vi "Autonomous Independent.vi"() -> ()   [LabVIEW 2016]
doc: "This VI is called when autonomous begins, and will automatically be terminated when autonomous ends. You can carry out timed or sensor driven robot movement independently without needing to return to the caller."
uses:
  <vilib>/Rock Robotics/WPI/Solenoid/WPI_SolenoidValue.ctl
  <vilib>/Rock Robotics/Network Tables/NT Read String.vi
  Robot Global Data.vi
  <vilib>/Rock Robotics/WPI/Solenoid/WPI_SolenoidSetEnum.vi
  <vilib>/Rock Robotics/WPI/Utilities/WPI_GetSetVariantRefNum.vi
  <vilib>/addons/control/pid/pid.llb/PID (DBL).vi
  <vilib>/addons/control/pid/NI_PID_pid.lvlib
panel:
  in  "Center":dbl=180.0 format="%#_13g"
  in  "MOE":dbl=25.0 format="%#_13g"
  in  "Speed 2":dbl=0.45 format="%#_13g"
  in  "PID gains L":T1={"proportional gain (Kc)"=1.5e-05, "integral time (Ti, min)"=1e-07, "derivative time (Td, min)"=0.0} {"derivative time (Td, min)" format="%.3f"; "integral time (Ti, min)" format="%.6f"; "proportional gain (Kc)" format="%.6f"}
  in  "PID gains R":T1={"proportional gain (Kc)"=1.5e-05, "integral time (Ti, min)"=1e-07, "derivative time (Td, min)"=0.0} {"derivative time (Td, min)" format="%.3f"; "integral time (Ti, min)" format="%.6f"; "proportional gain (Kc)" format="%.6f"}
  in  "Range":cluster{"output high":dbl, "output low":dbl}={"output high"=1.0, "output low"=-1.0} {"output low" format="%.2f"; "output high" format="%.2f"}
  out "Right V":cluster{"output":dbl, dbl, "Numeric":dbl}(graph)
  out "Left V":cluster{"output":dbl, dbl, "Numeric":dbl}(graph)
  in  "Speed":dbl=1.0 format="%#_13g"
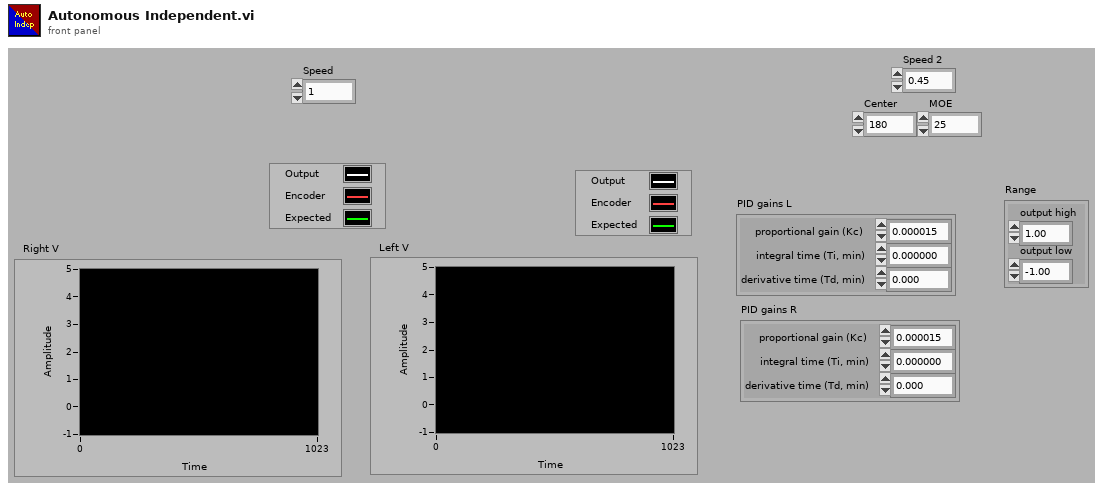
[diagram p1: front panel]
types:
  T1 = cluster{"proportional gain (Kc)":dbl, "integral time (Ti, min)":dbl, "derivative time (Td, min)":dbl}
  T2 = typedef "WPI_SolenoidValue.ctl" = enum16{"Off", "On", "Forward", "Reverse"}
  T3 = typedef "WPI_SolenoidDevRef.ctl" = cluster{"DevStatus":errorcluster, "Pneumatics Control Module":u8, "Forward Solenoid Channel":T4, "Reverse Solenoid Channel":T4}
  T4 = typedef "WPI_SolenoidChannel.ctl" = enum8{"Solenoid 0", "Solenoid 1", "Solenoid 2", "Solenoid 3", "Solenoid 4", "Solenoid 5", "Solenoid 6", "Solenoid 7", "Invalid"}
  T5 = typedef "WPI_RobotDriveDevRef.ctl" = cluster{"DevStatus":errorcluster, "Motors[]":T6[], "Square Inputs":bool, "Max Output":dbl}
  T6 = typedef "WPI_MotorControlDeviceRef.ctl" = cluster{"DeviceStatus":errorcluster, "Type":T7, "PWM":cluster{"PWM Channel":T8, "DeadBand":T9}, "CAN":cluster{"Device Number":u8, "SetOutput VI Ref":variant, "GetOutput VI Ref":variant, "Enable VI Ref":variant, "Disable VI Ref":variant, "Data":variant}, "Invert":bool}
  T7 = typedef "WPI_MotorControlType.ctl" = enum16{"PWM", "CAN"}
  T8 = typedef "FPGA_DIOPWMChannel.ctl" = enum8{"PWM 0", "PWM 1", "PWM 2", "PWM 3", "PWM 4", "PWM 5", "PWM 6", "PWM 7", "PWM 8", "PWM 9", "PWM MXP 0", "PWM MXP 1", "PWM MXP 2", "PWM MXP 3", "PWM MXP 4", "PWM MXP 5", "PWM MXP 6", "PWM MXP 7", "PWM MXP 8", "PWM MXP 9", "Invalid"}
  T9 = typedef "WPI_PWMDeadband.ctl" = cluster{"Name":string, "maxPositivePwm":i32, "minPositivePwm":i32, "centerPwm":i32, "maxNegativePwm":i32, "minNegativePwm":i32, "angularRange":u16}
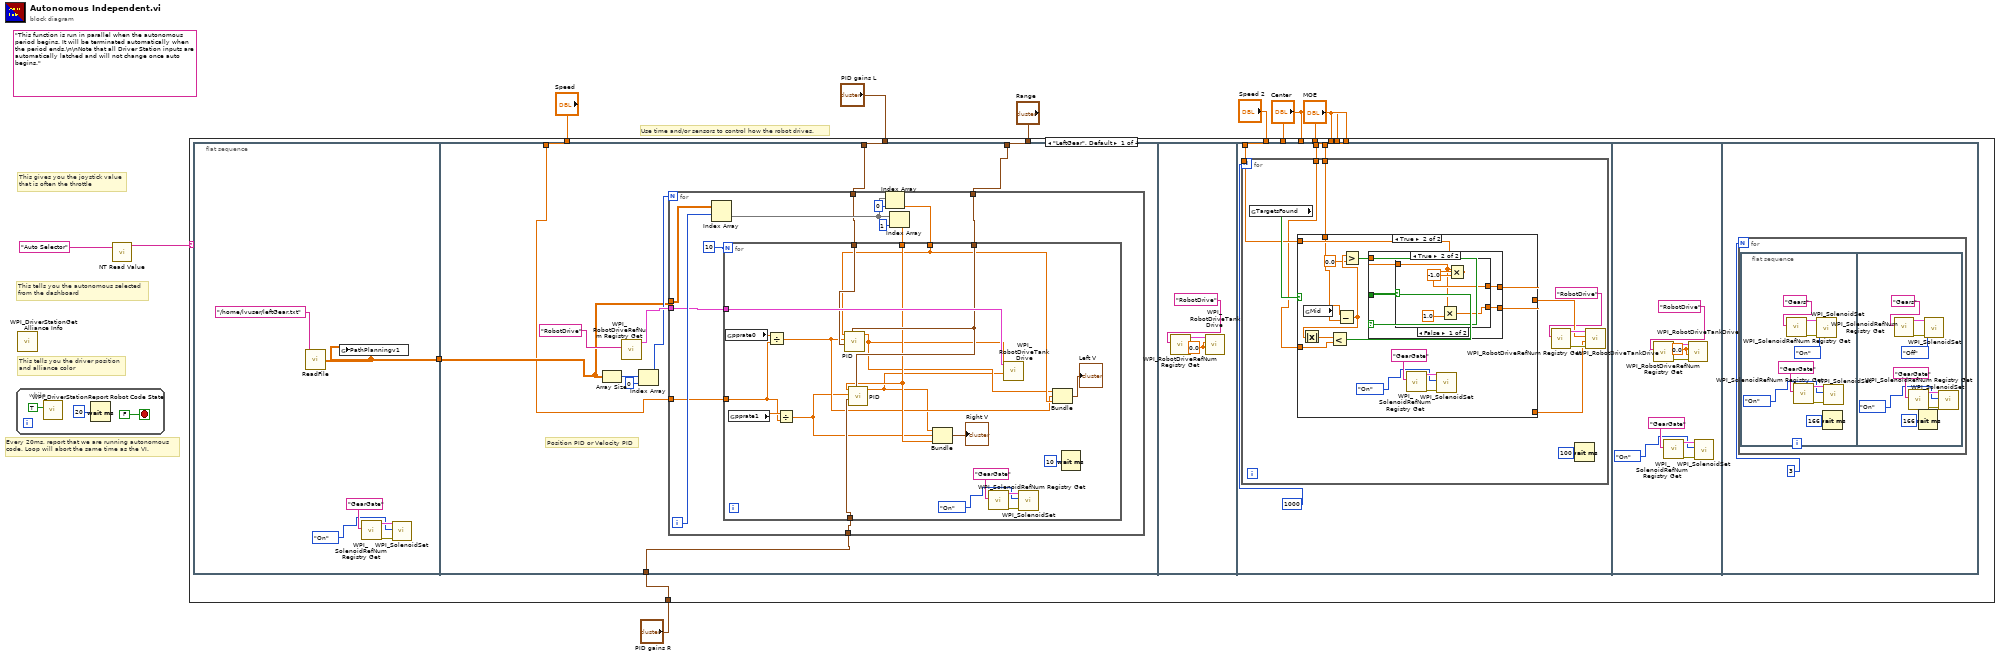
[diagram p0: block diagram]
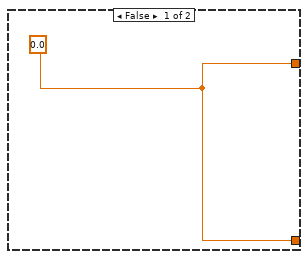
[diagram p2: hidden frame]
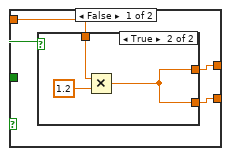
[diagram p3: hidden frame]
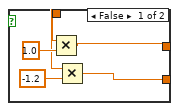
[diagram p4: hidden frame]
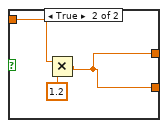
[diagram p5: hidden frame]
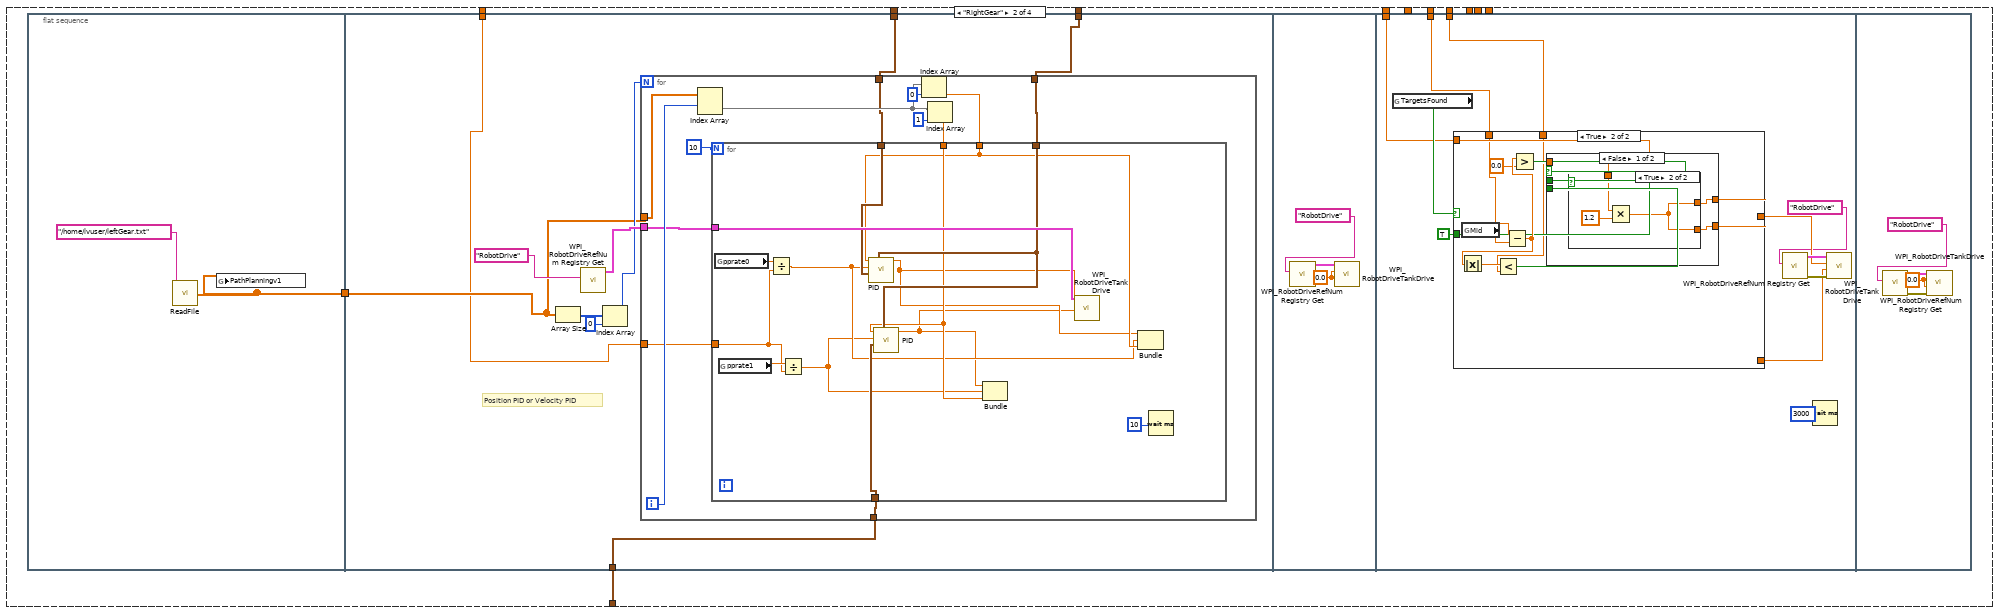
[diagram p6: hidden frame]
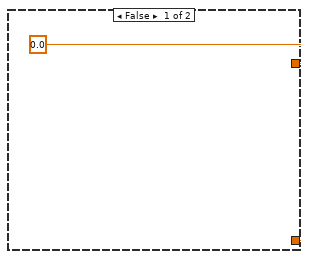
[diagram p7: hidden frame]
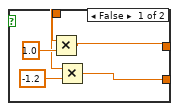
[diagram p8: hidden frame]
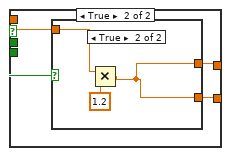
[diagram p9: hidden frame]
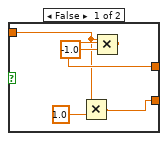
[diagram p10: hidden frame]
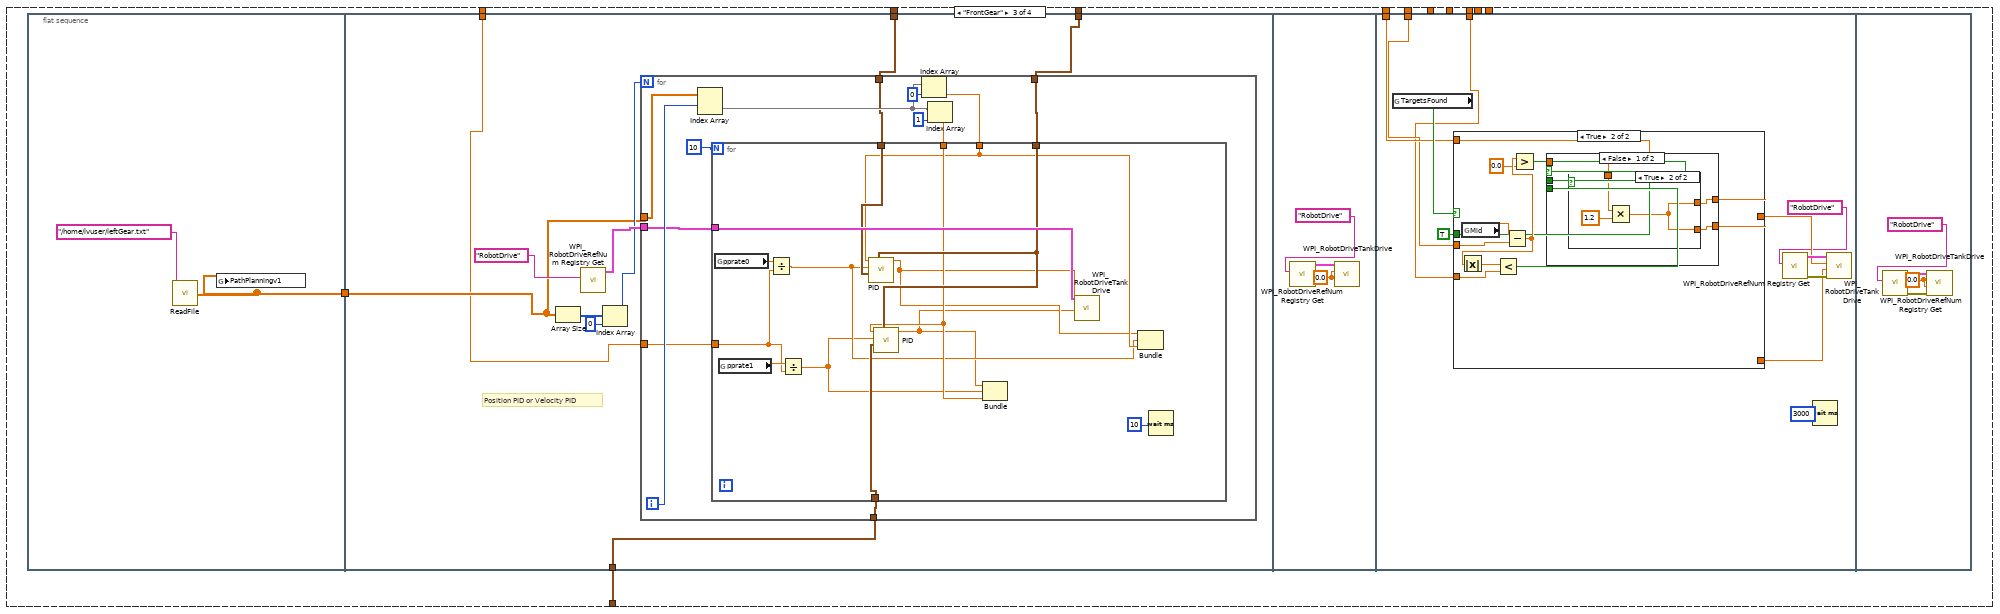
[diagram p11: hidden frame]
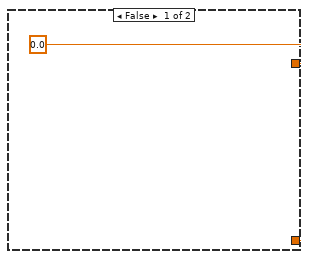
[diagram p12: hidden frame]
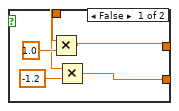
[diagram p13: hidden frame]
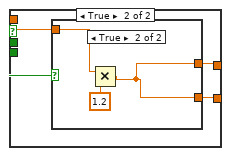
[diagram p14: hidden frame]
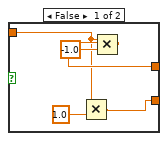
[diagram p15: hidden frame]
diagram:
  (unwired) "This function is run in parallel when the autonomous period begins. It will be terminated automatically when the period ends.\n\nNote that all Driver Station inputs are automatically latched and will not change once auto begins."
  # "This tells you the autonomous selected\nfrom the dashboard"
  # "Every 20ms, report that we are running autonomous\ncode. Loop will abort the same time as the VI."
  # "This gives you the joystick value\nthat is often the throttle"
  # "Use time and/or sensors to control how the robot drives."
  # "This tells you the driver position\nand alliance color"
  n1 = while {
    stop <- FALSE stop-if-true
    n2 = call <vilib>:"WPI_DriverStationReport Robot Code State.vi"("Autonomous"=TRUE) -> ()  [unwired: 10 in, 1 out]
    n3 = Wait (ms)(milliseconds to wait=u32 20) -> ()  [unwired: 1 out]
  }
  n4 = call <vilib>:"WPI_DriverStationGet Alliance Info.vi"() -> ()  [unwired: 12 out]
  n5 = call-poly <vilib>:"NT Read Value.vi"("Name"="Auto Selector") -> ("String"=w8:string)  [unwired: 9 in, 1 out]
  n6 = case shown="\"LeftGear\", Default" w8 {
    tunnel: "Range" -> [w19 w160 w262 _]
    tunnel: "PID gains L" -> [w18 w159 w261 _]
    tunnel: "Speed 2" -> [w17 w157 w260 _]
    tunnel: "Center" -> [w16 _ _ _]
    tunnel: "MOE" -> [w15 _ _ _]
    tunnel: "Speed" -> [w14 w158 w257 _]
    tunnel: "Center" -> [_ w156 _ _]
    tunnel: "MOE" -> [_ w155 _ _]
    tunnel: "Center" -> [_ _ w259 _]
    tunnel: "MOE" -> [_ _ w258 _]
    tunnel: "PID gains R" -> [w13 w154 w256 _]
    frame "LeftGear", Default {
      n7 = flat-sequence {
        tunnel: [w25] -> w20
        tunnel: w20 -> [w31]
        tunnel: w19 -> [w30]
        tunnel: w18 -> [w29]
        tunnel: w14 -> [w28]
        tunnel: w13 -> [w27]
        tunnel: w17 -> [w76]
        tunnel: w16 -> [w75]
        tunnel: w15 -> [w74]
        frame #0 {
          n8 = call "ReadFile.vi"("Name"="/home/lvuser/leftGear.txt") -> ("Array - Numeric"=w25:dbl[][])
          n9 = global write "Robot Global Data.vi" "PathPlanningv1"(w25) -> ()
          n10 = call <vilib>:"WPI_SolenoidRefNum Registry Get.vi"("refnum name"="GearGate") -> ("error out"=w24:errorcluster, "SolenoidDevRef"=w23:T3)  [unwired: 9 in]
          n11 = call-poly <vilib>:"WPI_SolenoidSet.vi"("error in (no error)"=w24, "Value"=WPI_SolenoidValue."On", "SolenoidDevRef"=w23) -> ()  [unwired: 7 in, 2 out]
        }
        frame #1 {
          # "Position PID or Velocity PID"
          n12 = Array Size(array=w31) -> (size(s)=w36:i32[])
          n13 = call <vilib>:"WPI_RobotDriveRefNum Registry Get.vi"("refnum name"="RobotDrive") -> ("RobotDriveDevRef"=w33:T5)  [unwired: 9 in, 1 out]
          n14 = Index Array(array=w36, index=0) -> (element=w32:i32)
          n15 = for {
            N: w32 -> [_]
            tunnel: w31 -> [w46]
            tunnel: w27 -> [w41]
            tunnel: w29 -> [w40]
            tunnel: w30 -> [w39]
            tunnel: w33 -> [w38]
            tunnel: w28 -> [w37]
            i -> [w43]
            n16 = Index Array(array=w46, index (row)=w43) -> (element=w49:dbl[])  [unwired: 1 in]
            n17 = Index Array(array=w49, index=0) -> (element=w45:dbl)
            n18 = Index Array(array=w49, index=1) -> (element=w44:dbl)
            n19 = for {
              N: 10 -> [_]
              tunnel: w45 -> [w63]
              tunnel: w44 -> [w64]
              tunnel: w41 -> [w67]
              tunnel: w40 -> [w66]
              tunnel: w39 -> [w65]
              tunnel: w38 -> [w68]
              tunnel: w37 -> [w56]
              n20 = global read "Robot Global Data.vi" "pprate0"() -> (w60:dbl)
              n21 = global read "Robot Global Data.vi" "pprate1"() -> (w57:dbl)
              n22 = Divide(x=w60, y=w56) -> (x/y=w59:dbl)
              n23 = Divide(x=w57, y=w56) -> (x/y=w58:dbl)
              n24 = call-poly <vilib>:"PID.vi"("output range"=w65, "PID gains"=w66, "process variable"=w59, "setpoint"=w63) -> ("output"=w55:dbl)  [unwired: 6 in, 1 out]
              n25 = call-poly <vilib>:"PID.vi"("output range"=w65, "PID gains"=w67, "process variable"=w58, "setpoint"=w64) -> ("output"=w54:dbl)  [unwired: 6 in, 1 out]
              n26 = Bundle("output"=w54, w58, "Numeric"=w64) -> (→"Right V":cluster{"output":dbl, dbl, "Numeric":dbl})  [unwired: 1 in]
              n27 = call <vilib>:"WPI_SolenoidRefNum Registry Get.vi"("refnum name"="GearGate") -> ("error out"=w53:errorcluster, "SolenoidDevRef"=w52:T3)  [unwired: 9 in]
              n28 = call <vilib>:"WPI_RobotDriveTankDrive.vi"("Right axis value"=w54, "Left axis value"=w55, "RobotDriveDevRef"=w68) -> ()  [unwired: 6 in, 3 out]
              n29 = call-poly <vilib>:"WPI_SolenoidSet.vi"("error in (no error)"=w53, "Value"=WPI_SolenoidValue."On", "SolenoidDevRef"=w52) -> ()  [unwired: 7 in, 2 out]
              n30 = Bundle("output"=w55, w59, "Numeric"=w63) -> (→"Left V":cluster{"output":dbl, dbl, "Numeric":dbl})  [unwired: 1 in]
              n31 = Wait (ms)(milliseconds to wait=10) -> ()  [unwired: 1 out]
            }
          }
        }
        frame #2 {
          w71 = 0.0 ("Right axis value")
          n32 = call <vilib>:"WPI_RobotDriveRefNum Registry Get.vi"("refnum name"="RobotDrive") -> ("RobotDriveDevRef"=w72:T5)  [unwired: 9 in, 1 out]
          n33 = call <vilib>:"WPI_RobotDriveTankDrive.vi"("Right axis value"=w71, "Left axis value"=w71, "RobotDriveDevRef"=w72) -> ()  [unwired: 6 in, 3 out]
        }
        frame #3 {
          n34 = for {
            N: 1000 -> [_]
            tunnel: w76 -> [w79]
            tunnel: w75 -> [w78]
            tunnel: w74 -> [w77]
            n35 = global read "Robot Global Data.vi" "TargetsFound"() -> (w80:bool)
            n36 = case shown="True" w80 {
              tunnel: [w87 w99] -> w83
              tunnel: [w87 w98] -> w84
              tunnel: w79 -> [_ w94]
              tunnel: w78 -> [_ w93]
              tunnel: w77 -> [_ w92]
              frame False {
                w87 = 0.0
              }
              frame True {
                n37 = global read "Robot Global Data.vi" "Mid"() -> (w102:dbl)
                n38 = Subtract(x=w102, y=w93) -> (x-y=w96:dbl)
                n39 = Absolute Value(x=w96) -> (abs(x)=w101:dbl)
                n40 = Less?(x=w101, y=w92) -> (x < y?=w100:bool)
                n41 = Greater?(x=w96, y=0.0) -> (0:w97:bool)
                n42 = case shown="True" w97 {
                  tunnel: w100 -> [w103 w118]
                  tunnel: [w104 w116] -> w99
                  tunnel: [w105 w117] -> w98
                  tunnel: w94 -> [w106 w115]
                  frame False {
                    n43 = case shown="True" w103 {
                      tunnel: [w111 w114] -> w105
                      tunnel: [w109 w114] -> w104
                      tunnel: w106 -> [w107 w112]
                      frame False {
                        n44 = Multiply(x=w107, y=1.0) -> (x*y=w111:dbl)
                        n45 = Multiply(x=w107, y=-1.2) -> (x*y=w109:dbl)
                      }
                      frame True {
                        n46 = Multiply(x=w112, y=1.2) -> (x*y=w114:dbl)
                      }
                    }
                  }
                  frame True {
                    n47 = case shown="False" w118 {
                      tunnel: [w123 w126] -> w117
                      tunnel: [w121 w126] -> w116
                      tunnel: w115 -> [w119 w124]
                      frame False {
                        n48 = Multiply(x=w119, y=1.0) -> (x*y=w121:dbl)
                        n49 = Multiply(x=w119, y=-1.0) -> (x*y=w123:dbl)
                      }
                      frame True {
                        n50 = Multiply(x=w124, y=1.2) -> (x*y=w126:dbl)
                      }
                    }
                  }
                }
                n51 = call <vilib>:"WPI_SolenoidRefNum Registry Get.vi"("refnum name"="GearGate") -> ("error out"=w91:errorcluster, "SolenoidDevRef"=w90:T3)  [unwired: 9 in]
                n52 = call-poly <vilib>:"WPI_SolenoidSet.vi"("error in (no error)"=w91, "Value"=WPI_SolenoidValue."On", "SolenoidDevRef"=w90) -> ()  [unwired: 7 in, 2 out]
              }
            }
            n53 = call <vilib>:"WPI_RobotDriveRefNum Registry Get.vi"("refnum name"="RobotDrive") -> ("error out"=w85:errorcluster, "RobotDriveDevRef"=w86:T5)  [unwired: 9 in]
            n54 = Wait (ms)(milliseconds to wait=100) -> ()  [unwired: 1 out]
            n55 = call <vilib>:"WPI_RobotDriveTankDrive.vi"("error in (no error)"=w85, "Right axis value"=w83, "Left axis value"=w84, "RobotDriveDevRef"=w86) -> ()  [unwired: 5 in, 3 out]
          }
        }
        frame #4 {
          w132 = 0.0 ("Left axis value")
          n56 = call <vilib>:"WPI_RobotDriveRefNum Registry Get.vi"("refnum name"="RobotDrive") -> ("error out"=w133:errorcluster, "RobotDriveDevRef"=w134:T5)  [unwired: 9 in]
          n57 = call <vilib>:"WPI_SolenoidRefNum Registry Get.vi"("refnum name"="GearGate") -> ("error out"=w130:errorcluster, "SolenoidDevRef"=w129:T3)  [unwired: 9 in]
          n58 = call <vilib>:"WPI_RobotDriveTankDrive.vi"("error in (no error)"=w133, "Right axis value"=w132, "Left axis value"=w132, "RobotDriveDevRef"=w134) -> ()  [unwired: 5 in, 3 out]
          n59 = call-poly <vilib>:"WPI_SolenoidSet.vi"("error in (no error)"=w130, "Value"=WPI_SolenoidValue."On", "SolenoidDevRef"=w129) -> ()  [unwired: 7 in, 2 out]
        }
        frame #5 {
          n60 = for {
            N: 3 -> [_]
            n61 = flat-sequence {
              frame #0 {
                n62 = call <vilib>:"WPI_SolenoidRefNum Registry Get.vi"("refnum name"="Gears") -> ("error out"=w144:errorcluster, "SolenoidDevRef"=w143:T3)  [unwired: 9 in]
                n63 = call <vilib>:"WPI_SolenoidRefNum Registry Get.vi"("refnum name"="GearGate") -> ("error out"=w139:errorcluster, "SolenoidDevRef"=w138:T3)  [unwired: 9 in]
                n64 = call-poly <vilib>:"WPI_SolenoidSet.vi"("error in (no error)"=w144, "Value"=WPI_SolenoidValue."On", "SolenoidDevRef"=w143) -> ()  [unwired: 7 in, 2 out]
                n65 = Wait (ms)(milliseconds to wait=166) -> ()  [unwired: 1 out]
                n66 = call-poly <vilib>:"WPI_SolenoidSet.vi"("error in (no error)"=w139, "Value"=WPI_SolenoidValue."On", "SolenoidDevRef"=w138) -> ()  [unwired: 7 in, 2 out]
              }
              frame #1 {
                n67 = call <vilib>:"WPI_SolenoidRefNum Registry Get.vi"("refnum name"="Gears") -> ("error out"=w153:errorcluster, "SolenoidDevRef"=w152:T3)  [unwired: 9 in]
                n68 = call <vilib>:"WPI_SolenoidRefNum Registry Get.vi"("refnum name"="GearGate") -> ("error out"=w148:errorcluster, "SolenoidDevRef"=w147:T3)  [unwired: 9 in]
                n69 = Wait (ms)(milliseconds to wait=166) -> ()  [unwired: 1 out]
                n70 = call-poly <vilib>:"WPI_SolenoidSet.vi"("error in (no error)"=w153, "Value"=WPI_SolenoidValue."Off", "SolenoidDevRef"=w152) -> ()  [unwired: 7 in, 2 out]
                n71 = call-poly <vilib>:"WPI_SolenoidSet.vi"("error in (no error)"=w148, "Value"=WPI_SolenoidValue."On", "SolenoidDevRef"=w147) -> ()  [unwired: 7 in, 2 out]
              }
            }
          }
        }
      }
    }
    frame "RightGear" {
      n72 = flat-sequence {
        tunnel: [w162] -> w161
        tunnel: w161 -> [w168]
        tunnel: w160 -> [w167]
        tunnel: w159 -> [w166]
        tunnel: w158 -> [w165]
        tunnel: w154 -> [w164]
        tunnel: w157 -> [w206]
        tunnel: w156 -> [w205]
        tunnel: w155 -> [w204]
        frame #0 {
          n73 = call "ReadFile.vi"("Name"="/home/lvuser/leftGear.txt") -> ("Array - Numeric"=w162:dbl[][])
          n74 = global write "Robot Global Data.vi" "PathPlanningv1"(w162) -> ()
        }
        frame #1 {
          # "Position PID or Velocity PID"
          n75 = Array Size(array=w168) -> (size(s)=w173:i32[])
          n76 = call <vilib>:"WPI_RobotDriveRefNum Registry Get.vi"("refnum name"="RobotDrive") -> ("RobotDriveDevRef"=w170:T5)  [unwired: 9 in, 1 out]
          n77 = Index Array(array=w173, index=0) -> (element=w169:i32)
          n78 = for {
            N: w169 -> [_]
            tunnel: w168 -> [w183]
            tunnel: w164 -> [w178]
            tunnel: w166 -> [w177]
            tunnel: w167 -> [w176]
            tunnel: w170 -> [w175]
            tunnel: w165 -> [w174]
            i -> [w180]
            n79 = Index Array(array=w183, index (row)=w180) -> (element=w186:dbl[])  [unwired: 1 in]
            n80 = Index Array(array=w186, index=0) -> (element=w182:dbl)
            n81 = Index Array(array=w186, index=1) -> (element=w181:dbl)
            n82 = for {
              N: 10 -> [_]
              tunnel: w182 -> [w194]
              tunnel: w181 -> [w195]
              tunnel: w178 -> [w198]
              tunnel: w177 -> [w197]
              tunnel: w176 -> [w196]
              tunnel: w175 -> [w199]
              tunnel: w174 -> [w189]
              n83 = global read "Robot Global Data.vi" "pprate0"() -> (w193:dbl)
              n84 = global read "Robot Global Data.vi" "pprate1"() -> (w190:dbl)
              n85 = Divide(x=w193, y=w189) -> (x/y=w192:dbl)
              n86 = Divide(x=w190, y=w189) -> (x/y=w191:dbl)
              n87 = call-poly <vilib>:"PID.vi"("output range"=w196, "PID gains"=w197, "process variable"=w192, "setpoint"=w194) -> ("output"=w188:dbl)  [unwired: 6 in, 1 out]
              n88 = call-poly <vilib>:"PID.vi"("output range"=w196, "PID gains"=w198, "process variable"=w191, "setpoint"=w195) -> ("output"=w187:dbl)  [unwired: 6 in, 1 out]
              n89 = Bundle("output"=w187, w191, "Numeric"=w195) -> ()  [unwired: 1 in, 1 out]
              n90 = call <vilib>:"WPI_RobotDriveTankDrive.vi"("Right axis value"=w187, "Left axis value"=w188, "RobotDriveDevRef"=w199) -> ()  [unwired: 6 in, 3 out]
              n91 = Bundle("output"=w188, w192, "Numeric"=w194) -> ()  [unwired: 1 in, 1 out]
              n92 = Wait (ms)(milliseconds to wait=10) -> ()  [unwired: 1 out]
            }
          }
        }
        frame #2 {
          w202 = 0.0 ("Right axis value")
          n93 = call <vilib>:"WPI_RobotDriveRefNum Registry Get.vi"("refnum name"="RobotDrive") -> ("RobotDriveDevRef"=w203:T5)  [unwired: 9 in, 1 out]
          n94 = call <vilib>:"WPI_RobotDriveTankDrive.vi"("Right axis value"=w202, "Left axis value"=w202, "RobotDriveDevRef"=w203) -> ()  [unwired: 6 in, 3 out]
        }
        frame #3 {
          n95 = global read "Robot Global Data.vi" "TargetsFound"() -> (w207:bool)
          n96 = case shown="True" w207 {
            tunnel: [w215 w224] -> w210
            tunnel: [w215 w223] -> w211
            tunnel: TRUE -> [_ w219]
            tunnel: w206 -> [_ w218]
            tunnel: w205 -> [_ w217]
            tunnel: w204 -> [_ w216]
            frame False {
              w215 = 0.0
            }
            frame True {
              n97 = global read "Robot Global Data.vi" "Mid"() -> (w227:dbl)
              n98 = Subtract(x=w227, y=w217) -> (x-y=w221:dbl)
              n99 = Absolute Value(x=w221) -> (abs(x)=w226:dbl)
              n100 = Less?(x=w226, y=w216) -> (x < y?=w225:bool)
              n101 = Greater?(x=w221, y=0.0) -> (0:w222:bool)
              n102 = case shown="False" w222 {
                tunnel: w225 -> [w228 w243]
                tunnel: [w229 w241] -> w224
                tunnel: [w230 w242] -> w223
                tunnel: w219 -> [_ _]
                tunnel: w218 -> [w231 w240]
                frame False {
                  n103 = case shown="True" w228 {
                    tunnel: [w236 w239] -> w230
                    tunnel: [w234 w239] -> w229
                    tunnel: w231 -> [w232 w237]
                    frame False {
                      n104 = Multiply(x=w232, y=1.0) -> (x*y=w236:dbl)
                      n105 = Multiply(x=w232, y=-1.2) -> (x*y=w234:dbl)
                    }
                    frame True {
                      n106 = Multiply(x=w237, y=1.2) -> (x*y=w239:dbl)
                    }
                  }
                }
                frame True {
                  n107 = case shown="True" w243 {
                    tunnel: [w248 w251] -> w242
                    tunnel: [w246 w251] -> w241
                    tunnel: w240 -> [w244 w249]
                    frame False {
                      n108 = Multiply(x=w244, y=1.0) -> (x*y=w246:dbl)
                      n109 = Multiply(x=w244, y=-1.0) -> (x*y=w248:dbl)
                    }
                    frame True {
                      n110 = Multiply(x=w249, y=1.2) -> (x*y=w251:dbl)
                    }
                  }
                }
              }
            }
          }
          n111 = call <vilib>:"WPI_RobotDriveRefNum Registry Get.vi"("refnum name"="RobotDrive") -> ("error out"=w212:errorcluster, "RobotDriveDevRef"=w213:T5)  [unwired: 9 in]
          n112 = Wait (ms)(milliseconds to wait=3000) -> ()  [unwired: 1 out]
          n113 = call <vilib>:"WPI_RobotDriveTankDrive.vi"("error in (no error)"=w212, "Right axis value"=w210, "Left axis value"=w211, "RobotDriveDevRef"=w213) -> ()  [unwired: 5 in, 3 out]
        }
        frame #4 {
          w253 = 0.0 ("Left axis value")
          n114 = call <vilib>:"WPI_RobotDriveRefNum Registry Get.vi"("refnum name"="RobotDrive") -> ("error out"=w254:errorcluster, "RobotDriveDevRef"=w255:T5)  [unwired: 9 in]
          n115 = call <vilib>:"WPI_RobotDriveTankDrive.vi"("error in (no error)"=w254, "Right axis value"=w253, "Left axis value"=w253, "RobotDriveDevRef"=w255) -> ()  [unwired: 5 in, 3 out]
        }
      }
    }
    frame "FrontGear" {
      n116 = flat-sequence {
        tunnel: [w264] -> w263
        tunnel: w263 -> [w270]
        tunnel: w262 -> [w269]
        tunnel: w261 -> [w268]
        tunnel: w257 -> [w267]
        tunnel: w256 -> [w266]
        tunnel: w260 -> [w308]
        tunnel: w259 -> [w307]
        tunnel: w258 -> [w306]
        frame #0 {
          n117 = call "ReadFile.vi"("Name"="/home/lvuser/leftGear.txt") -> ("Array - Numeric"=w264:dbl[][])
          n118 = global write "Robot Global Data.vi" "PathPlanningv1"(w264) -> ()
        }
        frame #1 {
          # "Position PID or Velocity PID"
          n119 = Array Size(array=w270) -> (size(s)=w275:i32[])
          n120 = call <vilib>:"WPI_RobotDriveRefNum Registry Get.vi"("refnum name"="RobotDrive") -> ("RobotDriveDevRef"=w272:T5)  [unwired: 9 in, 1 out]
          n121 = Index Array(array=w275, index=0) -> (element=w271:i32)
          n122 = for {
            N: w271 -> [_]
            tunnel: w270 -> [w285]
            tunnel: w266 -> [w280]
            tunnel: w268 -> [w279]
            tunnel: w269 -> [w278]
            tunnel: w272 -> [w277]
            tunnel: w267 -> [w276]
            i -> [w282]
            n123 = Index Array(array=w285, index (row)=w282) -> (element=w288:dbl[])  [unwired: 1 in]
            n124 = Index Array(array=w288, index=0) -> (element=w284:dbl)
            n125 = Index Array(array=w288, index=1) -> (element=w283:dbl)
            n126 = for {
              N: 10 -> [_]
              tunnel: w284 -> [w296]
              tunnel: w283 -> [w297]
              tunnel: w280 -> [w300]
              tunnel: w279 -> [w299]
              tunnel: w278 -> [w298]
              tunnel: w277 -> [w301]
              tunnel: w276 -> [w291]
              n127 = global read "Robot Global Data.vi" "pprate0"() -> (w295:dbl)
              n128 = global read "Robot Global Data.vi" "pprate1"() -> (w292:dbl)
              n129 = Divide(x=w295, y=w291) -> (x/y=w294:dbl)
              n130 = Divide(x=w292, y=w291) -> (x/y=w293:dbl)
              n131 = call-poly <vilib>:"PID.vi"("output range"=w298, "PID gains"=w299, "process variable"=w294, "setpoint"=w296) -> ("output"=w290:dbl)  [unwired: 6 in, 1 out]
              n132 = call-poly <vilib>:"PID.vi"("output range"=w298, "PID gains"=w300, "process variable"=w293, "setpoint"=w297) -> ("output"=w289:dbl)  [unwired: 6 in, 1 out]
              n133 = Bundle("output"=w289, w293, "Numeric"=w297) -> ()  [unwired: 1 in, 1 out]
              n134 = call <vilib>:"WPI_RobotDriveTankDrive.vi"("Right axis value"=w289, "Left axis value"=w290, "RobotDriveDevRef"=w301) -> ()  [unwired: 6 in, 3 out]
              n135 = Bundle("output"=w290, w294, "Numeric"=w296) -> ()  [unwired: 1 in, 1 out]
              n136 = Wait (ms)(milliseconds to wait=10) -> ()  [unwired: 1 out]
            }
          }
        }
        frame #2 {
          w304 = 0.0 ("Right axis value")
          n137 = call <vilib>:"WPI_RobotDriveRefNum Registry Get.vi"("refnum name"="RobotDrive") -> ("RobotDriveDevRef"=w305:T5)  [unwired: 9 in, 1 out]
          n138 = call <vilib>:"WPI_RobotDriveTankDrive.vi"("Right axis value"=w304, "Left axis value"=w304, "RobotDriveDevRef"=w305) -> ()  [unwired: 6 in, 3 out]
        }
        frame #3 {
          n139 = global read "Robot Global Data.vi" "TargetsFound"() -> (w309:bool)
          n140 = case shown="True" w309 {
            tunnel: [w317 w326] -> w312
            tunnel: [w317 w325] -> w313
            tunnel: TRUE -> [_ w321]
            tunnel: w308 -> [_ w320]
            tunnel: w307 -> [_ w319]
            tunnel: w306 -> [_ w318]
            frame False {
              w317 = 0.0
            }
            frame True {
              n141 = global read "Robot Global Data.vi" "Mid"() -> (w329:dbl)
              n142 = Subtract(x=w329, y=w319) -> (x-y=w323:dbl)
              n143 = Absolute Value(x=w323) -> (abs(x)=w328:dbl)
              n144 = Less?(x=w328, y=w318) -> (x < y?=w327:bool)
              n145 = Greater?(x=w323, y=0.0) -> (0:w324:bool)
              n146 = case shown="False" w324 {
                tunnel: w327 -> [w330 w345]
                tunnel: [w331 w343] -> w326
                tunnel: [w332 w344] -> w325
                tunnel: w321 -> [_ _]
                tunnel: w320 -> [w333 w342]
                frame False {
                  n147 = case shown="True" w330 {
                    tunnel: [w338 w341] -> w332
                    tunnel: [w336 w341] -> w331
                    tunnel: w333 -> [w334 w339]
                    frame False {
                      n148 = Multiply(x=w334, y=1.0) -> (x*y=w338:dbl)
                      n149 = Multiply(x=w334, y=-1.2) -> (x*y=w336:dbl)
                    }
                    frame True {
                      n150 = Multiply(x=w339, y=1.2) -> (x*y=w341:dbl)
                    }
                  }
                }
                frame True {
                  n151 = case shown="True" w345 {
                    tunnel: [w350 w353] -> w344
                    tunnel: [w348 w353] -> w343
                    tunnel: w342 -> [w346 w351]
                    frame False {
                      n152 = Multiply(x=w346, y=1.0) -> (x*y=w348:dbl)
                      n153 = Multiply(x=w346, y=-1.0) -> (x*y=w350:dbl)
                    }
                    frame True {
                      n154 = Multiply(x=w351, y=1.2) -> (x*y=w353:dbl)
                    }
                  }
                }
              }
            }
          }
          n155 = call <vilib>:"WPI_RobotDriveRefNum Registry Get.vi"("refnum name"="RobotDrive") -> ("error out"=w314:errorcluster, "RobotDriveDevRef"=w315:T5)  [unwired: 9 in]
          n156 = Wait (ms)(milliseconds to wait=3000) -> ()  [unwired: 1 out]
          n157 = call <vilib>:"WPI_RobotDriveTankDrive.vi"("error in (no error)"=w314, "Right axis value"=w312, "Left axis value"=w313, "RobotDriveDevRef"=w315) -> ()  [unwired: 5 in, 3 out]
        }
        frame #4 {
          w355 = 0.0 ("Left axis value")
          n158 = call <vilib>:"WPI_RobotDriveRefNum Registry Get.vi"("refnum name"="RobotDrive") -> ("error out"=w356:errorcluster, "RobotDriveDevRef"=w357:T5)  [unwired: 9 in]
          n159 = call <vilib>:"WPI_RobotDriveTankDrive.vi"("error in (no error)"=w356, "Right axis value"=w355, "Left axis value"=w355, "RobotDriveDevRef"=w357) -> ()  [unwired: 5 in, 3 out]
        }
      }
    }
    frame "Nothing" {
    }
  }
